vi "TCP-receiver.vi"() -> ()   [LabVIEW 2020]
panel:
  out "Waveform Chart":i32(graph)
  out "Gauge":dbl(knob) scale=0.0..100.0
  out "number":i32
  in  "stop":bool
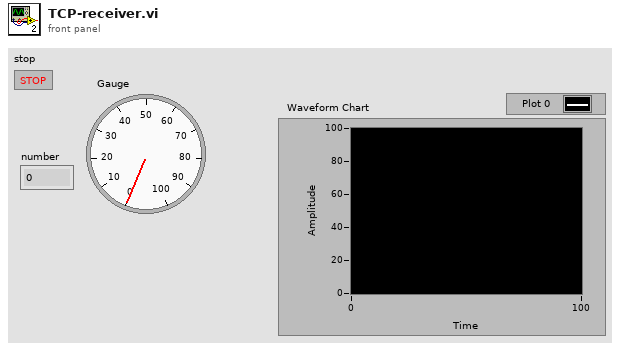
[diagram p1: front panel]
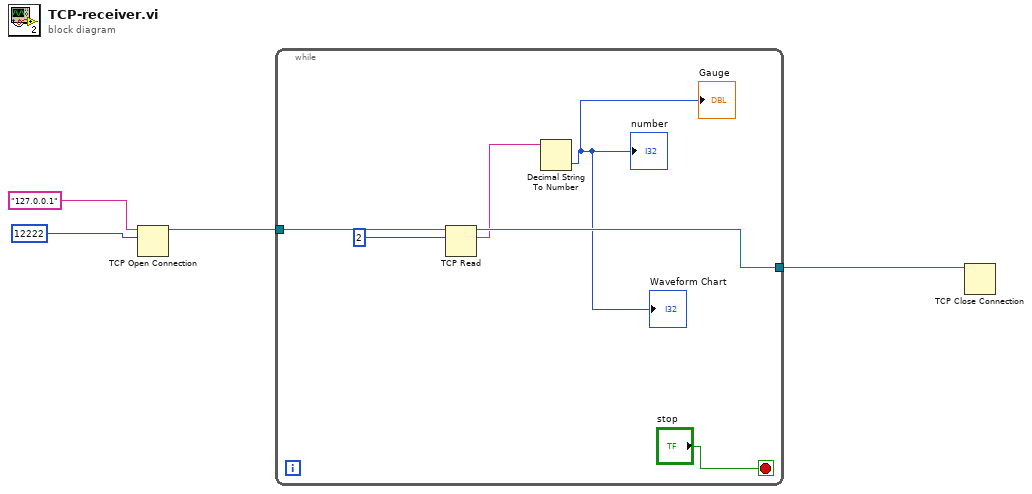
[diagram p0: block diagram]
diagram:
  n1 = TCP Open Connection(address="127.0.0.1", remote port or service name=12222) -> (connection ID=w2:refnum<k5>)  [unwired: 3 in, 1 out]
  n2 = while {
    tunnel: w2 -> [w10]
    tunnel: [w8] -> w1
    stop <- "stop" stop-if-true
    n3 = TCP Read(connection ID=w10, bytes to read=2) -> (connection ID out=w8:refnum<k5>, data out=w6:string)  [unwired: 3 in, 1 out]
    n4 = Decimal String To Number(string=w6) -> (number=→"number" →"Gauge" →"Waveform Chart":i32)  [unwired: 2 in, 1 out]
  }
  n5 = TCP Close Connection(connection ID=w1) -> ()  [unwired: 2 in, 2 out]
